vi "Frame Decoder.vi"(8 "error in (no error)":errorcluster, 10 "Frame Data":u8[](array[numeric]), 11 "Frame Detail":string[][](array[string])) -> (0 "error out":errorcluster, 2 "Raw Data":u64[](array[numeric]), 3 "Frame Detail With Value":string[](array[string]))   [LabVIEW 2023]
uses:
  <vilib>/Utility/error.llb/Trim Whitespace One-Sided.vi
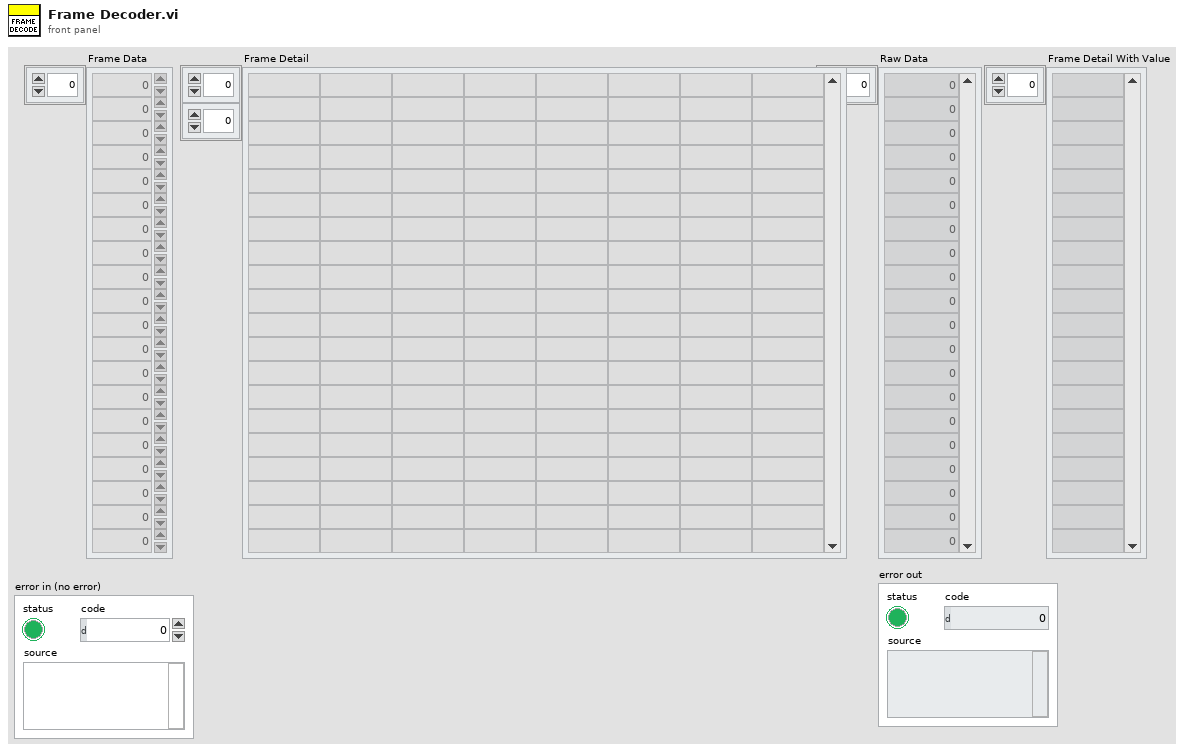
[diagram p1: front panel]
types:
  T1 = enum16{"big-endian, network order", "native, host order", "little-endian"}
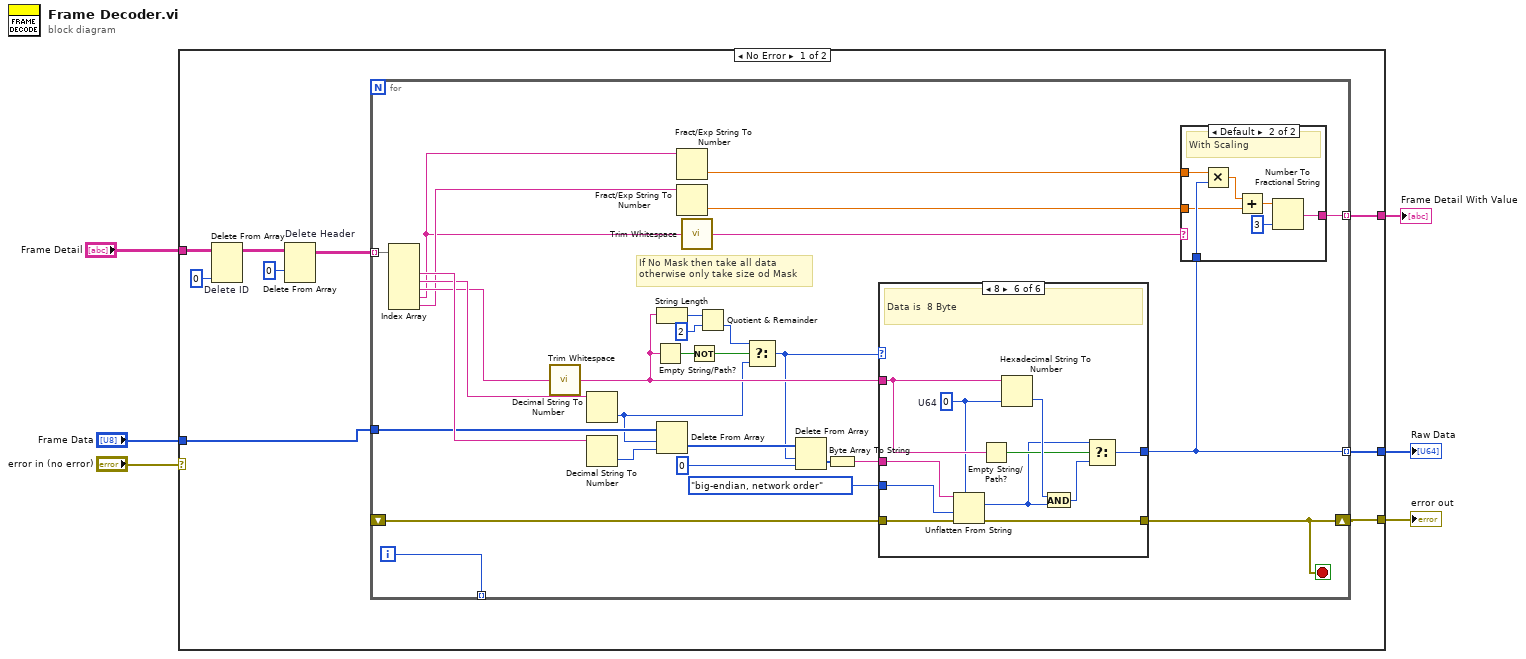
[diagram p0: block diagram]
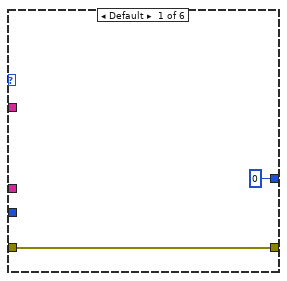
[diagram p2: hidden frame]
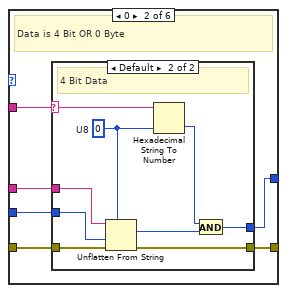
[diagram p3: hidden frame]
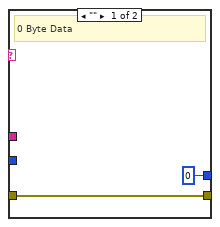
[diagram p4: hidden frame]
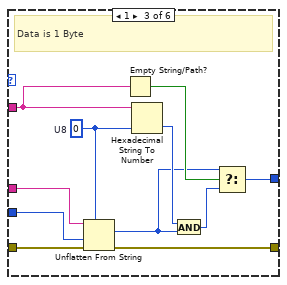
[diagram p5: hidden frame]
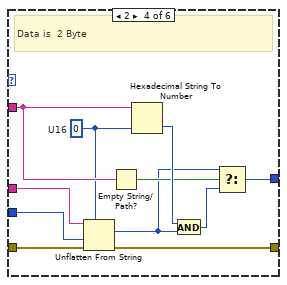
[diagram p6: hidden frame]
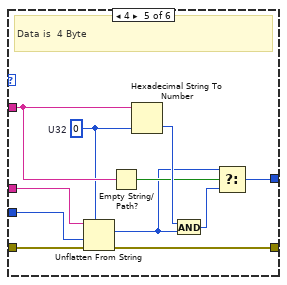
[diagram p7: hidden frame]
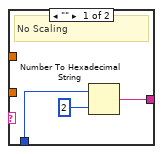
[diagram p8: hidden frame]
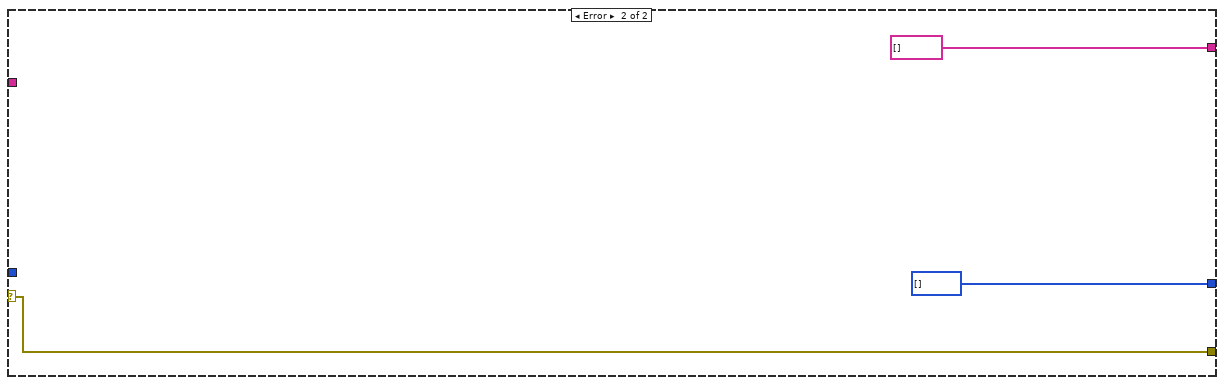
[diagram p9: hidden frame]
diagram:
  n1 = case shown="No Error" "error in (no error)" {
    selector: "error in (no error)" -> [_ w120]
    tunnel: "Frame Detail" -> [w15 _]
    tunnel: [w10 w120] -> w2
    tunnel: [w9 string[] []] -> w3
    tunnel: "Frame Data" -> [w8 _]
    tunnel: [w7 u8[] [] ("ResponseData")] -> w6
    frame No Error {
      n2 = Delete From Array "Delete ID"(array=w15, index (col)=0 ("disabled index (col)")) -> (array with subset deleted=w12:string[][])  [unwired: 2 in, 1 out]
      n3 = Delete From Array "Delete Header"(array=w12, index (row)=0) -> (array with subset deleted=w14:string[][])  [unwired: 2 in, 1 out]
      n4 = for {
        tunnel: w14 -> [w44] mode=indexing
        tunnel: w8 -> [w41]
        tunnel: [w31] -> _ mode=indexing
        shift-right: [w28] -> w10
        shift-left: _ -> [w29]
        tunnel: [w27] -> w9 mode=indexing
        tunnel: [w16] -> w7 mode=indexing
        i -> [w31]
        stop <- w28 stop-if-true
        # "If No Mask then take all data\notherwise only take size od Mask"
        n5 = Index Array(array=w44) -> (element #2=w43:string, element #3=w42:string, element #4=w39:string, element #5=w33:string, element #6=w37:string)  [unwired: 6 in, 1 out]
        n6 = call <vilib>:"Trim Whitespace.vi"("string"=w39) -> ("trimmed string"=w23:string)  [unwired: 1 in]
        n7 = Decimal String To Number(string=w42) -> (number=w20:i32)  [unwired: 2 in, 1 out]
        n8 = Decimal String To Number(string=w43) -> (number=w40:i32)  [unwired: 2 in, 1 out]
        n9 = Empty String/Path?(string/path=w23) -> (empty?=w22:bool)
        n10 = String Length(string=w23) -> (length=w32:i32)
        n11 = Delete From Array(array=w41, length=w20, index=w40) -> (deleted portion=w38:u8[])  [unwired: 1 out]
        n12 = Fract/Exp String To Number(string=w33) -> (number=w36:dbl)  [unwired: 3 in, 1 out]
        n13 = Fract/Exp String To Number(string=w37) -> (number=w35:dbl)  [unwired: 3 in, 1 out]
        n14 = call <vilib>:"Trim Whitespace.vi"("string"=w33) -> ("trimmed string"=w34:string)  [unwired: 1 in]
        n15 = Not(x=w22) -> (.not. x?=w19:bool)
        n16 = Quotient & Remainder(x=w32, y=2) -> (floor(x/y)=w21:i32)  [unwired: 1 out]
        n17 = Select(t=w21, s=w19, f=w20) -> (s? t:f=w17:i32)
        n18 = Delete From Array(array=w38, length=w17, index=0) -> (deleted portion=w25:u8[])  [unwired: 1 out]
        n19 = Byte Array To String(unsigned byte array=w25) -> (string=w18:string)
        n20 = case shown="8" w17 {
          tunnel: T1."big-endian, network order" ("byte order (0:big-endian, network order)") -> [_ w52 w74 w85 w96 w107]
          tunnel: w29 -> [w46 w51 w73 w84 w95 w106]
          tunnel: [w46 w50 w72 w83 w94 w105] -> w28
          tunnel: w23 -> [_ w49 w71 w82 w93 w104]
          tunnel: [u8 0 ("U8") w47 w67 w78 w89 w100] -> w16
          tunnel: w18 -> [_ w48 w66 w77 w88 w99]
          frame Default {
          }
          frame 0 {
            # "Data is 4 Bit OR 0 Byte"
            n21 = case shown="Default" w49 {
              selector: w49 -> [_ w60]
              tunnel: w52 -> [_ w63]
              tunnel: w51 -> [w53 w62]
              tunnel: [w53 w61] -> w50
              tunnel: w48 -> [_ w58]
              tunnel: [u8 0 w55] -> w47
              frame "" {
                # "0 Byte Data"
              }
              frame Default {
                w56 = u8 0  # U8
                # "4 Bit Data"
                n22 = Unflatten From String(type=w56, binary string=w58, byte order (0:big-endian, network order)=w63, error in (no error)=w62) -> (value=w57:u8, error out=w61:errorcluster)  [unwired: 1 in, 1 out]
                n23 = Hexadecimal String To Number(string=w60, default (0uL)=w56) -> (number=w59:u8)  [unwired: 1 in, 1 out]
                n24 = And(x=w59, y=w57) -> (x .and. y?=w55:u8)
              }
            }
          }
          frame 1 {
            w64 = u8 0  # U8
            # "Data is 1 Byte"
            n25 = Unflatten From String(type=w64, binary string=w66, byte order (0:big-endian, network order)=w74, error in (no error)=w73) -> (value=w65:u8, error out=w72:errorcluster)  [unwired: 1 in, 1 out]
            n26 = Empty String/Path?(string/path=w71) -> (empty?=w69:bool)
            n27 = Hexadecimal String To Number(string=w71, default (0uL)=w64) -> (number=w70:u8)  [unwired: 1 in, 1 out]
            n28 = And(x=w70, y=w65) -> (x .and. y?=w68:u8)
            n29 = Select(t=w65, s=w69, f=w68) -> (s? t:f=w67:u8)
          }
          frame 2 {
            w75 = u16 0  # U16
            # "Data is  2 Byte"
            n30 = Unflatten From String(type=w75, binary string=w77, byte order (0:big-endian, network order)=w85, error in (no error)=w84) -> (value=w76:u16, error out=w83:errorcluster)  [unwired: 1 in, 1 out]
            n31 = Empty String/Path?(string/path=w82) -> (empty?=w80:bool)
            n32 = Hexadecimal String To Number(string=w82, default (0uL)=w75) -> (number=w81:u16)  [unwired: 1 in, 1 out]
            n33 = And(x=w81, y=w76) -> (x .and. y?=w79:u16)
            n34 = Select(t=w76, s=w80, f=w79) -> (s? t:f=w78:u16)
          }
          frame 4 {
            w86 = u32 0  # U32
            # "Data is  4 Byte"
            n35 = Unflatten From String(type=w86, binary string=w88, byte order (0:big-endian, network order)=w96, error in (no error)=w95) -> (value=w87:u32, error out=w94:errorcluster)  [unwired: 1 in, 1 out]
            n36 = Empty String/Path?(string/path=w93) -> (empty?=w91:bool)
            n37 = Hexadecimal String To Number(string=w93, default (0uL)=w86) -> (number=w92:u32)  [unwired: 1 in, 1 out]
            n38 = And(x=w92, y=w87) -> (x .and. y?=w90:u32)
            n39 = Select(t=w87, s=w91, f=w90) -> (s? t:f=w89:u32)
          }
          frame 8 {
            w97 = u64 0  # U64
            # "Data is  8 Byte"
            n40 = Unflatten From String(type=w97, binary string=w99, byte order (0:big-endian, network order)=w107, error in (no error)=w106) -> (value=w98:u64, error out=w105:errorcluster)  [unwired: 1 in, 1 out]
            n41 = Empty String/Path?(string/path=w104) -> (empty?=w102:bool)
            n42 = Hexadecimal String To Number(string=w104, default (0uL)=w97) -> (number=w103:u64)  [unwired: 1 in, 1 out]
            n43 = And(x=w103, y=w98) -> (x .and. y?=w101:u64)
            n44 = Select(t=w98, s=w102, f=w101) -> (s? t:f=w100:u64)
          }
        }
        n45 = case shown="Default" w34 {
          tunnel: w16 -> [w109 w116]
          tunnel: w36 -> [_ w115]
          tunnel: w35 -> [_ w114]
          tunnel: [w108 w112] -> w27
          frame "" {
            # "No Scaling"
            n46 = Number To Hexadecimal String(1:i16 2 ("width (-)"), 2:w109) -> (0:w108:string)
          }
          frame Default {
            # "With Scaling"
            n47 = Multiply(x=w115, y=w116) -> (x*y=w117:dbl)
            n48 = Add(x=w117, y=w114) -> (x+y=w113:dbl)
            n49 = Number To Fractional String(number=w113, precision (6)=i16 3) -> (F-format string=w112:string)  [unwired: 2 in]
          }
        }
      }
    }
    frame Error {
    }
  }
  "Raw Data" <- w6
  "Frame Detail With Value" <- w3
  "error out" <- w2
